vi "Set Tree Data.vi"(10 "Tree Data":T1(array[cluster]), 11 "Executioner in":refnum<class "Executioner.lvclass">) -> (3 "Executioner out":refnum<class "Executioner.lvclass">)   [LabVIEW 2017, in "Test Executive.lvlib" / "Executioner.lvclass"]
uses:
  <vilib>/gpm_packages/@cs/test-executive/Source/Test Executive/Executioner/Executioner.lvclass
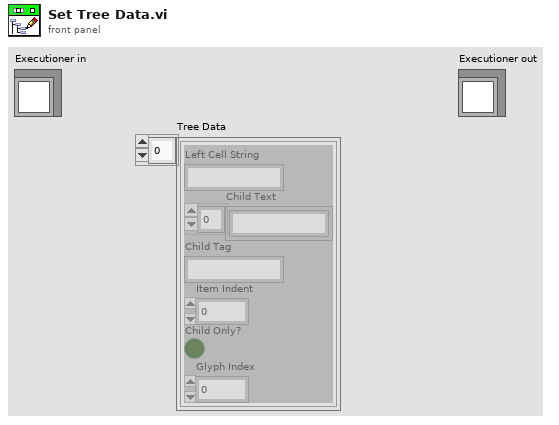
[diagram p1: front panel]
types:
  T1 = cluster{"Left Cell String":string, "Child Text":string[], "Child Tag":string, "Item Indent":i32, "Child Only?":bool, "Glyph Index":i32}[]
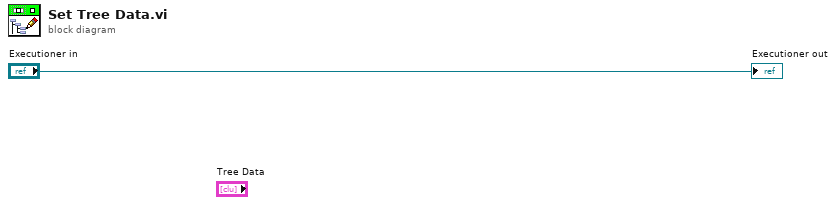
[diagram p0: block diagram]
diagram:
  "Executioner out" <- "Executioner in"
